vi "Periodic Tasks.vi"(8 "error in":errorcluster) -> ()   [LabVIEW 2018]
doc: "This VI runs in parallel to other tasks. It can contain as many user-defined periodic loops as you need. These can carry out PID or other sorts of timed response."
uses:
  DriveLoopEnum.ctl
  <vilib>/Rock Robotics/WPI/ThirdParty/Phoenix-LabVIEW/Motor Controller/Get/CTRE_Phoenix_MotorController_GetSelectedSensorData.vi
  <vilib>/Rock Robotics/WPI/ThirdParty/Phoenix-LabVIEW/Pigeon IMU/CTRE_PigeonIMU_GetFusedHeading.vi
  <vilib>/Rock Robotics/WPI/ThirdParty/Phoenix-LabVIEW/Pigeon IMU/CTRE_PigeonIMU_GetTempStateUpTime.vi
  driveShifterEnum.ctl
  <vilib>/Rock Robotics/WPI/ThirdParty/Phoenix-LabVIEW/Pigeon IMU/CTRE_PigeonIMU_PigeonState.ctl
  <vilib>/Rock Robotics/WPI/ThirdParty/Phoenix-LabVIEW/Pigeon IMU/CTRE_PigeonIMU_CalibrationMode.ctl
panel:
  out "XY Graph":cluster{dbl[], dbl[]}[](graph)
  out "Heading":dbl(graph)
  out "Temp/State/UpTime":T3 {"CurrentMode" items=["BootTareGryoAccel"=0, "Temperature"=1, "Magnetometer12Pt"=2, "Magnetometer360"=3, "Accelerometer"=5]}
  out "Fused Heading":T4
  out "Position (Raw Sensor Units) 2":i32
  out "Position (Raw Sensor Units)":i32
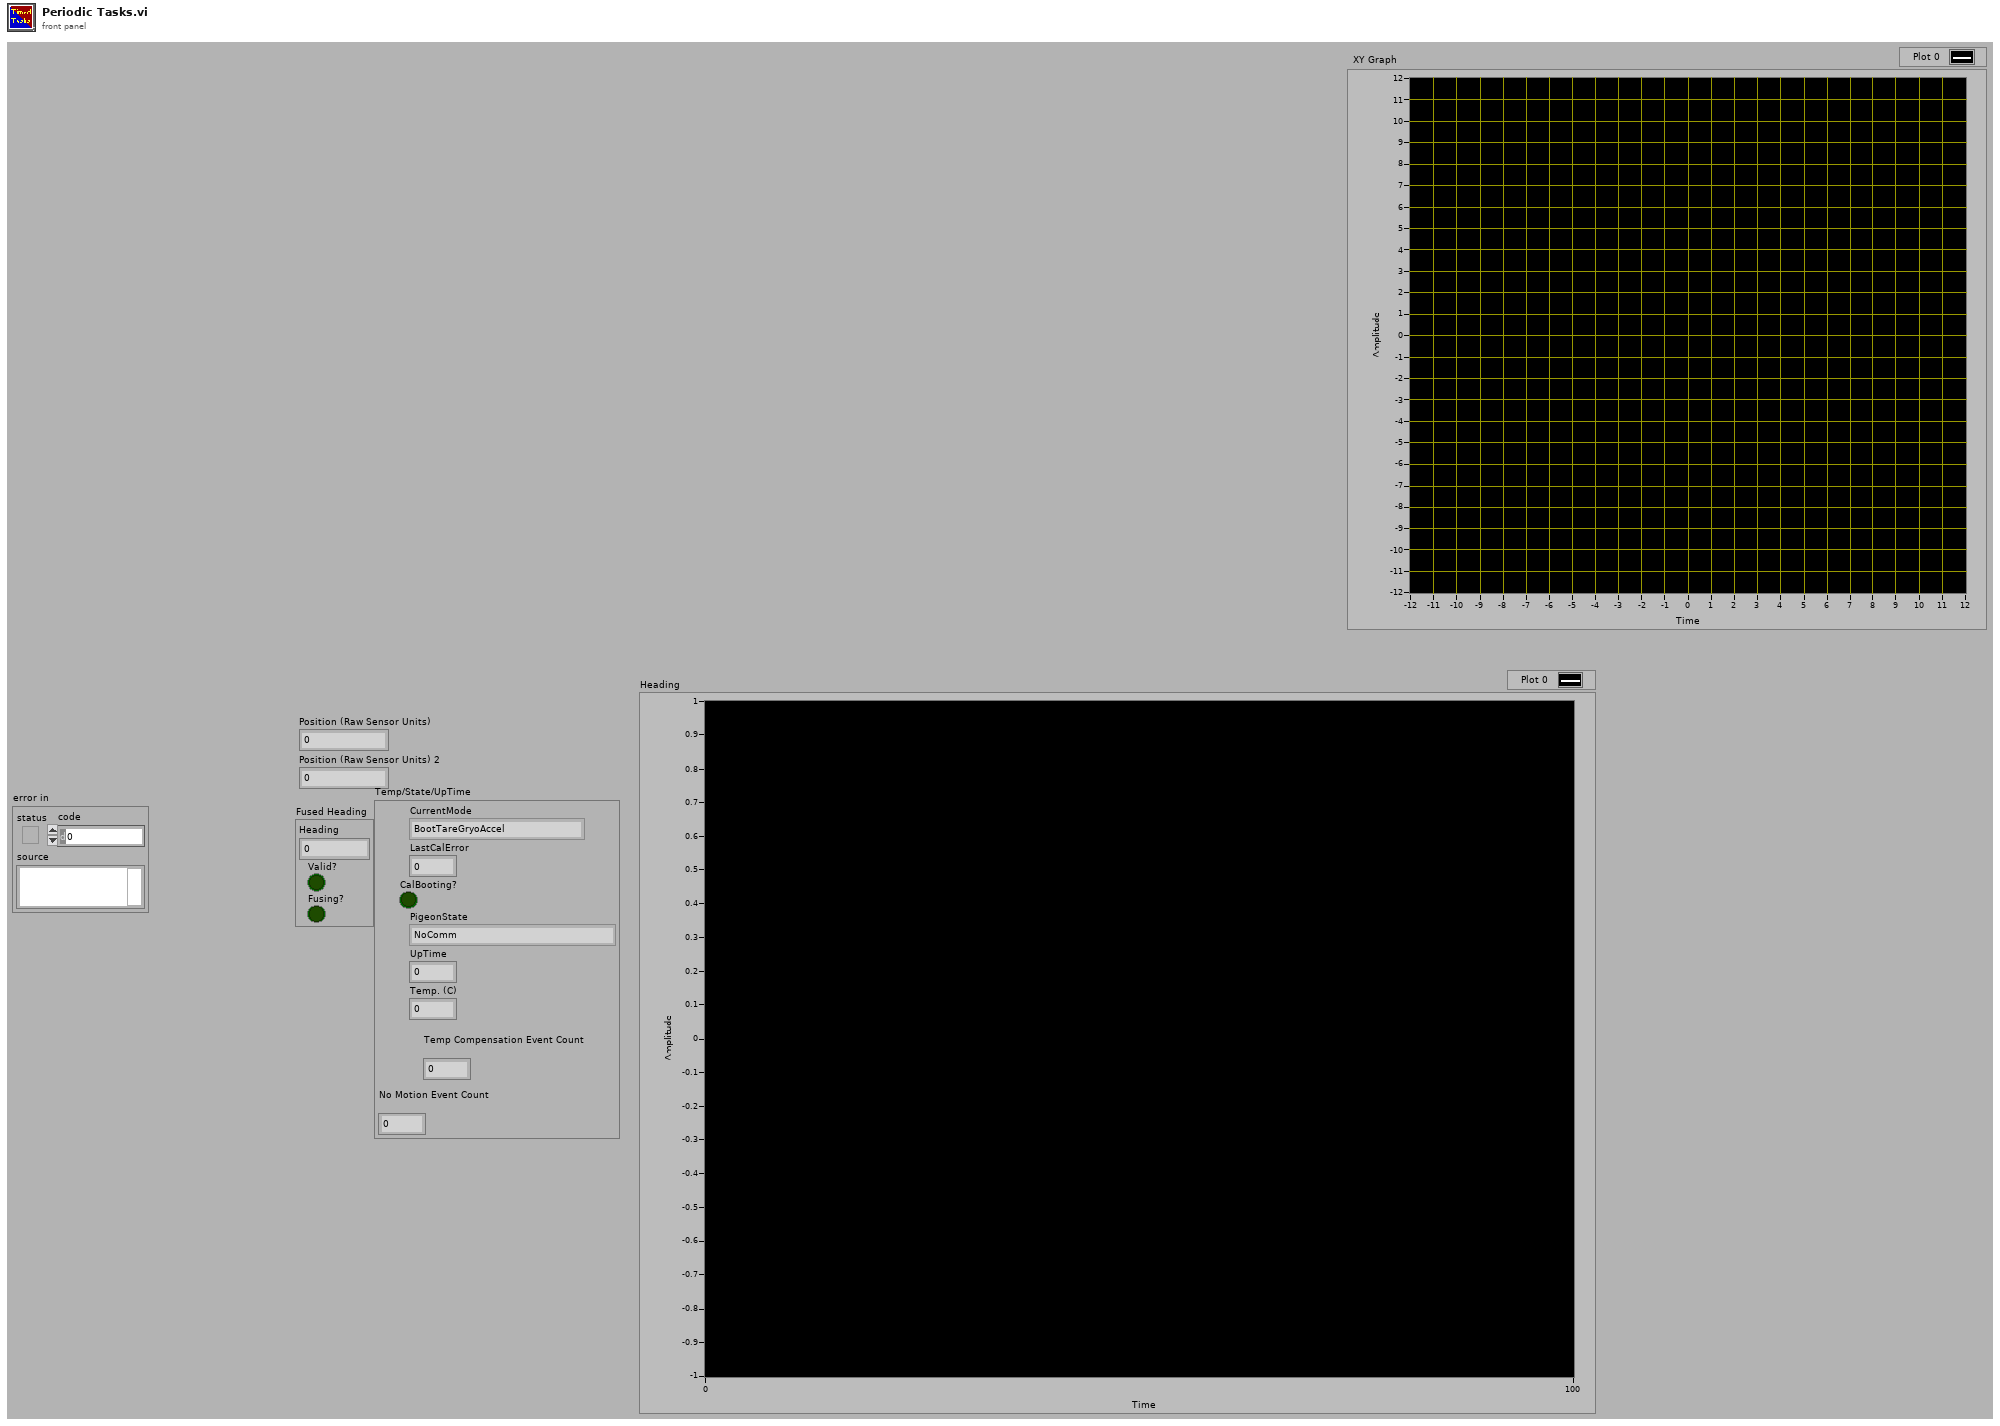
[diagram p1: front panel]
types:
  T1 = typedef "CTRE_PigeonIMU_CalibrationMode.ctl" = u16
  T2 = typedef "CTRE_PigeonIMU_PigeonState.ctl" = enum16{"NoComm", "Initializing", "Ready", "UserCalibration"}
  T3 = cluster{"CurrentMode":T1, "LastCalError":i32, "CalBooting?":bool, "PigeonState":T2, "UpTime":u32, "Temp. (C)":dbl, "Temp Compensation Event Count":u32, "No Motion Event Count":u32}
  T4 = cluster{"Heading":dbl, "Valid?":bool, "Fusing?":bool}
  T5 = typedef "DriveLoopEnum.ctl" = enum16{"Manual", "Motion Magic"}
  T6 = typedef "CTRE_PigeonIMU_DeviceRef.ctl" = cluster{"DeviceStatus":errorcluster, "Device Number":u8, "Type":T7, "Device ID":u32, "Handle":u64, "UsageFrame":u32, "Library Path":path}
  T7 = typedef "CTRE_PigeonIMU_ConnectionType.ctl" = u32
  T8 = typedef "WPI_MotorControlDeviceRef.ctl" = cluster{"DeviceStatus":errorcluster, "Type":T9, "PWM":cluster{"PWM Channel":T10, "DeadBand":T11}, "CAN":cluster{"Device Number":u8, "SetOutput VI Ref":variant, "GetOutput VI Ref":variant, "Enable VI Ref":variant, "Disable VI Ref":variant, "Data":variant}, "Invert":bool, "DIO PWM":cluster{"PWM \"Enable\" Channel":T10, "DIOChannel":T12, "PWM Rate":dbl}}
  T9 = typedef "WPI_MotorControlType.ctl" = enum16{"PWM", "CAN", "DIO PWM"}
  T10 = typedef "FPGA_DIOPWMChannel.ctl" = enum8{"PWM 0", "PWM 1", "PWM 2", "PWM 3", "PWM 4", "PWM 5", "PWM 6", "PWM 7", "PWM 8", "PWM 9", "PWM MXP 0", "PWM MXP 1", "PWM MXP 2", "PWM MXP 3", "PWM MXP 4", "PWM MXP 5", "PWM MXP 6", "PWM MXP 7", "PWM MXP 8", "PWM MXP 9", "Invalid"}
  T11 = typedef "WPI_PWMDeadband.ctl" = cluster{"Name":string, "maxPositivePwm":i32, "minPositivePwm":i32, "centerPwm":i32, "maxNegativePwm":i32, "minNegativePwm":i32, "angularRange":u16}
  T12 = typedef "FPGA_DIOChannel.ctl" = enum8{"DIO 0", "DIO 1", "DIO 2", "DIO 3", "DIO 4", "DIO 5", "DIO 6", "DIO 7", "DIO 8", "DIO 9", "DIO MXP 0", "DIO MXP 1", "DIO MXP 2", "DIO MXP 3", "DIO MXP 4", "DIO MXP 5", "DIO MXP 6", "DIO MXP 7", "DIO MXP 8", "DIO MXP 9", "DIO MXP 10", "DIO MXP 11", "DIO MXP 12", "DIO MXP 13", "DIO MXP 14", "DIO MXP 15", "SPI Port CS1", "SPI Port CS2", "SPI Port CS3", "SPI Port MISO", "SPI Port MOSI", "Invalid"}
  T13 = typedef "driveShifterEnum.ctl" = enum16{"Low", "High"}
  T14 = enum16{"Inches -> Sensor Units", "Sensor Units -> Inches"}
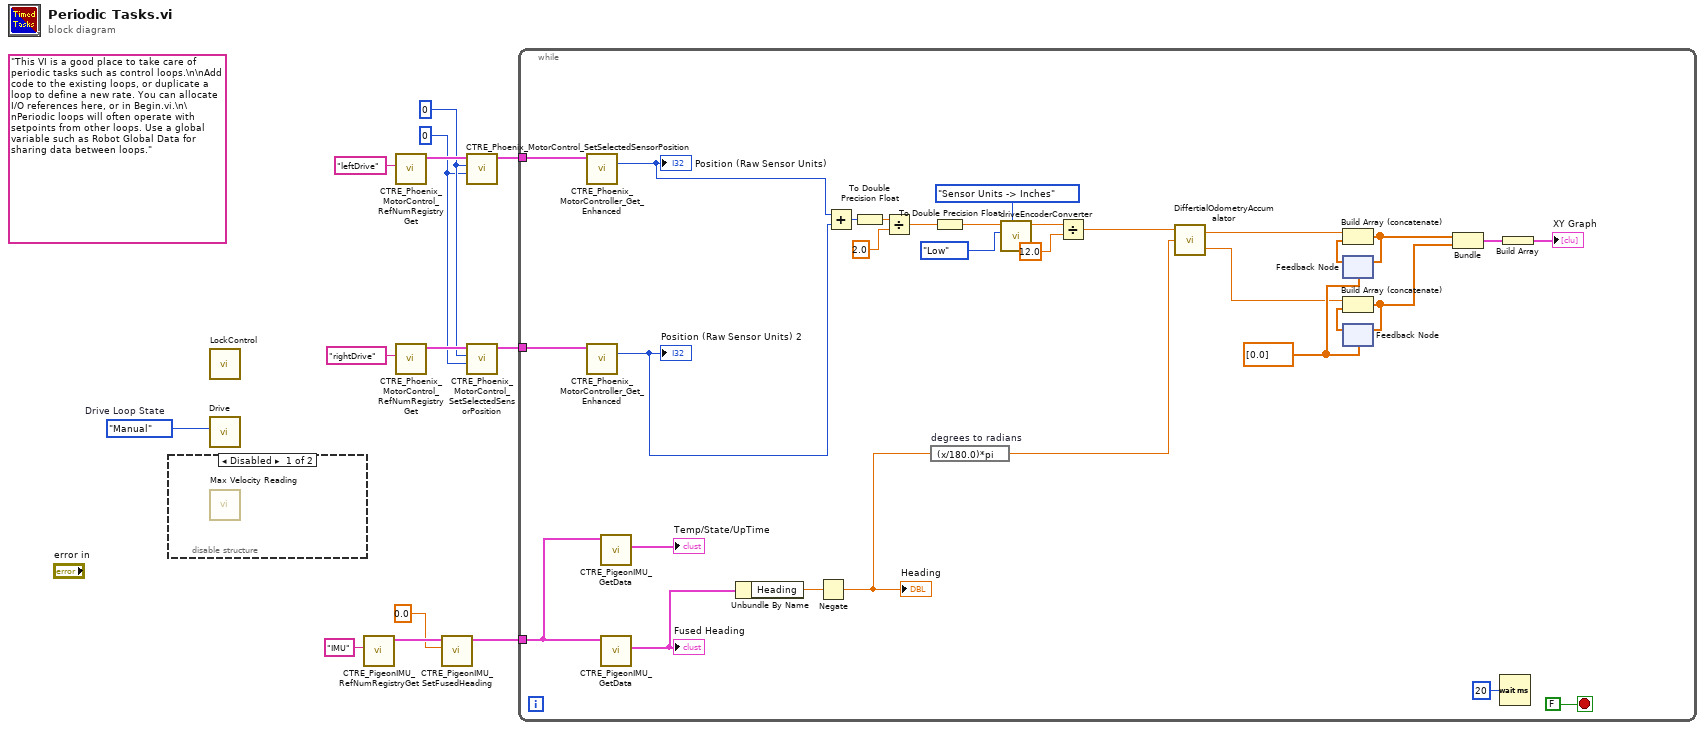
[diagram p0: block diagram]
diagram:
  w5 = u32 0 ("pidLoopIdx")
  w6 = 0 ("New Sensor Position")
  w13 = DriveLoopEnum."Manual"  # Drive Loop State
  (unwired) "This VI is a good place to take care of periodic tasks such as control loops.\n\nAdd code to the existing loops, or duplicate a loop to define a new rate. You can allocate I/O references here, or in Begin.vi.\n\nPeriodic loops will often operate with setpoints from other loops. Use a global variable such as Robot Global Data for sharing data between loops."
  n1 = disable-structure shown="Disabled" {
    frame Disabled {
      n2 = call "Max Velocity Reading.vi"() -> ()  [unwired: 12 in]
    }
    frame Enabled {
    }
  }
  n3 = call "LockControl.vi"() -> ()  [unwired: 12 in]
  n4 = call "Drive.vi"("Drive Loop State"=w13) -> ()  [unwired: 11 in]
  n5 = call <vilib>:"CTRE_PigeonIMU_RefNumRegistryGet.vi"("refnum name"="IMU") -> ("PigeonIMUDevRef"=w3:T6)  [unwired: 9 in, 1 out]
  n6 = call <vilib>:"CTRE_Phoenix_MotorControl_RefNumRegistryGet.vi"("refnum name"="leftDrive") -> ("PhoenixMotorControlDevRef"=w10:T8)  [unwired: 9 in, 1 out]
  n7 = call <vilib>:"CTRE_Phoenix_MotorControl_RefNumRegistryGet.vi"("refnum name"="rightDrive") -> ("PhoenixMotorControlDevRef"=w8:T8)  [unwired: 9 in, 1 out]
  n8 = call <vilib>:"CTRE_PigeonIMU_SetFusedHeading.vi"("Value"=0.0, "PigeonIMUDevRef 2"=w3) -> ("PigeonIMUDevRef"=w2:T6)  [unwired: 8 in, 1 out]
  n9 = call <vilib>:"CTRE_Phoenix_MotorControl_SetSelectedSensorPosition.vi"("pidLoopIdx"=w5, "New Sensor Position"=w6, "PhoenixMotorControlDevRef"=w10) -> ("PhoenixMotorControlDevRef"=w9:T8)  [unwired: 7 in, 1 out]
  n10 = call <vilib>:"CTRE_Phoenix_MotorControl_SetSelectedSensorPosition.vi"("pidLoopIdx"=w5, "New Sensor Position"=w6, "PhoenixMotorControlDevRef"=w8) -> ("PhoenixMotorControlDevRef"=w7:T8)  [unwired: 7 in, 1 out]
  n11 = while {
    tunnel: w9 -> [w42]
    tunnel: w7 -> [w41]
    tunnel: w2 -> [w40]
    stop <- FALSE stop-if-true
    w33 = dbl[] [0.0]
    n12 = call-poly <vilib>:"CTRE_Phoenix_MotorController_Get_Enhanced.vi"("PhoenixMotorControlDevRef"=w42) -> ("Position (Raw Sensor Units)"=w21:i32)  [unwired: 11 in, 3 out]
    "Position (Raw Sensor Units)" <- w21
    n13 = call-poly <vilib>:"CTRE_Phoenix_MotorController_Get_Enhanced.vi"("PhoenixMotorControlDevRef"=w41) -> ("Position (Raw Sensor Units)"=w26:i32)  [unwired: 11 in, 3 out]
    "Position (Raw Sensor Units) 2" <- w26
    n14 = call-poly <vilib>:"CTRE_PigeonIMU_GetData.vi"("PigeonIMUDevRef"=w40) -> ("Temp/State/UpTime"=→"Temp/State/UpTime":T3)  [unwired: 8 in, 2 out]
    n15 = call-poly <vilib>:"CTRE_PigeonIMU_GetData.vi"("PigeonIMUDevRef"=w40) -> ("Fused Heading"=w38:T4)  [unwired: 8 in, 2 out]
    "Fused Heading" <- w38
    n16 = Unbundle By Name(w38) -> ("Heading"=w31:dbl)
    n17 = Negate(x=w31) -> (-x=w18:dbl)
    "Heading" <- w18
    n18 = Add(x=w21, y=w26) -> (x+y=w25:i32)
    n19 = To Double Precision Float(number=w25) -> (double precision float=w23:dbl)
    n20 = Divide(x=w23, y=2.0) -> (x/y=w19:dbl)
    n21 = expression code="(x/180.0)*pi" "degrees to radians"(w18) -> (w16:dbl)
    n22 = To Double Precision Float(number=w19) -> (double precision float=w20:dbl)
    n23 = call "driveEncoderConverter.vi"("Conversion Direction"=T14."Sensor Units -> Inches", "Gear Setting"=driveShifterEnum."Low", "Input"=w20) -> ("Output"=w30:dbl)  [unwired: 8 in]
    n24 = Divide(x=w30, y=12.0) -> (x/y=w17:dbl)
    n25 = call "DiffertialOdometryAccumalator.vi"("Position"=w17, "Heading (rad)"=w16) -> ("X"=w15:dbl, "Y"=w14:dbl)  [unwired: 3 in]
    n26 = feedback #1(w33) -> (w34:dbl[])
    n27 = Build Array (concatenate)(w15, w34) -> (w36:dbl[])
    n28 = feedback-in #1(w36) -> ()
    n29 = feedback #2(w33) -> (w37:dbl[])
    n30 = Build Array (concatenate)(w14, w37) -> (w35:dbl[])
    n31 = feedback-in #2(w35) -> ()
    n32 = Bundle(w36, w35) -> (w22:cluster{dbl[], dbl[]})  [unwired: 1 in]
    n33 = Wait (ms)(milliseconds to wait=u32 20) -> ()  [unwired: 1 out]
    n34 = Build Array(w22) -> (→"XY Graph":cluster{dbl[], dbl[]}[])
  }
